vi "ApplyVIPC.vi"(8 "error in (no error)":errorcluster) -> (0 "error out":errorcluster)   [LabVIEW 2020, in "CICD.lvlib"]
doc: "Check currently installed packages and apply specified package if required."
uses:
  CICD.lvlib
  <vilib>/Wiresmith Technology/G CLI/CLI Class/CLI.lvclass
  <vilib>/Wiresmith Technology/G CLI/Argument Parser/Option Set Class/Option Set.lvclass
  <vilib>/Wiresmith Technology/G CLI/Argument Parser/Option Class/Argument Type.ctl
  <vilib>/Wiresmith Technology/G CLI/Argument Parser/Option Class/Option.lvclass
  <vilib>/Wiresmith Technology/G CLI/Argument Parser/Option Class/Option Configuration.ctl
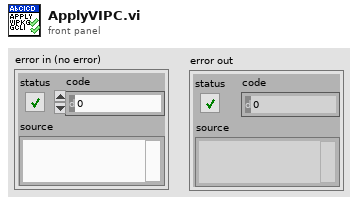
[diagram p1: front panel]
types:
  T1 = typedef "Option Parser.lvlib/Option.lvclass/Option Configuration.ctl" = cluster{"Option Type":T2, "Option Labels":string[], "Key":string, "Description":string, "Required":bool, "Default Value":string}
  T2 = typedef "Option Parser.lvlib/Option.lvclass/Argument Type.ctl" = enum16{"flag", "value"}
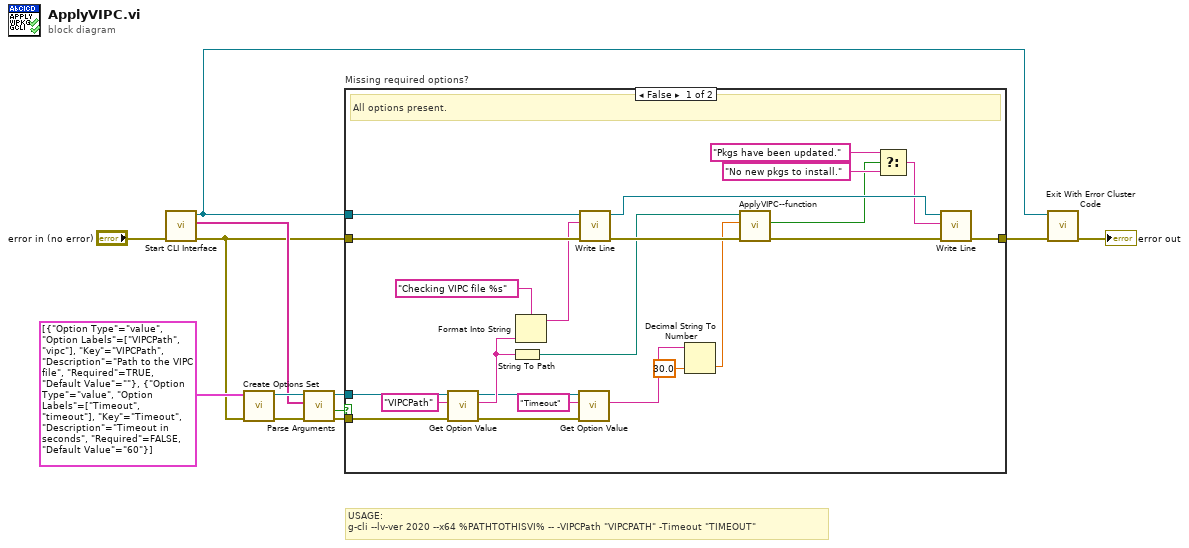
[diagram p0: block diagram]
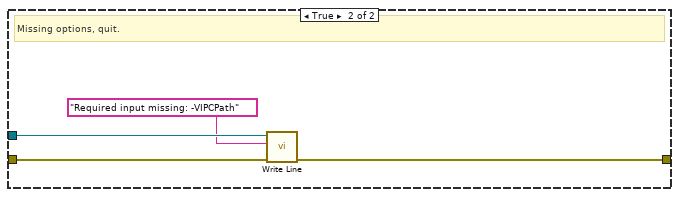
[diagram p2: hidden frame]
diagram:
  # "USAGE:\ng-cli --lv-ver 2020 --x64 %PATHTOTHISVI% -- -VIPCPath \"VIPCPATH\" -Timeout \"TIMEOUT\""
  n1 = call <vilib>:"Start CLI Interface.vi"("error in (no error)"="error in (no error)") -> ("error out"=w4:errorcluster, "Custom Parameters"=w8:string[], "CLI out"=w2:refnum<class "CLI.lvclass">)  [unwired: 7 in, 1 out]
  n2 = call <vilib>:"Create Options Set.vi"("error in (no error)"=w4, "Options"=T1[] [{"Option Type"=enum."value", "Option Labels"=["VIPCPath", "vipc"], "Key"="VIPCPath", "Description"="Path to the VIPC file", "Required"=TRUE, "Default Value"=""}, {"Option Type"=enum."value", "Option Labels"=["Timeout", "timeout"], "Key"="Timeout", "Description"="Timeout in seconds", "Required"=FALSE, "Default Value"="60"}]) -> ("error out"=w10:errorcluster, "Option Set out"=w11:refnum<class "Option Set.lvclass">)  [unwired: 8 in]
  n3 = call <vilib>:"Parse Arguments.vi"("error in (no error)"=w10, "Arguments"=w8, "Option Set in"=w11) -> ("error out"=w6:errorcluster, "Missing Options"=w5:bool, "Option Set out"=w7:refnum<class "Option Set.lvclass">)  [unwired: 5 in, 1 out]
  n4 = case "Missing required options?" shown="False" w5 {
    tunnel: w7 -> [w35 _]
    tunnel: w6 -> [w34 _]
    tunnel: w2 -> [w31 w38]
    tunnel: w4 -> [w32 w39]
    tunnel: [w20 w36] -> w3
    frame False {
      # "All options present."
      n5 = call <vilib>:"Get Option Value.vi"("error in (no error)"=w34, "Option Key"="VIPCPath", "Option Set in"=w35) -> ("error out"=w25:errorcluster, "Value"=w29:string, "Option Set out"=w26:refnum<class "Option Set.lvclass">)  [unwired: 5 in, 1 out]
      n6 = String To Path(string=w29) -> (path=w14:path)
      n7 = Format Into String(format string="Checking VIPC file %s" ("Text to Write"), w29) -> (resulting string=w28:string)  [unwired: 2 in, 1 out]
      n8 = call <vilib>:"Get Option Value.vi"("error in (no error)"=w25, "Option Key"="Timeout", "Option Set in"=w26) -> ("Value"=w22:string)  [unwired: 5 in, 3 out]
      n9 = call <vilib>:"Write Line.vi"("error in (no error)"=w32, "Text to Write"=w28, "CLI in"=w31) -> ("error out"=w27:errorcluster, "CLI out"=w19:refnum<class "CLI.lvclass">)  [unwired: 7 in]
      n10 = Decimal String To Number(string=w22, default (0L)=30.0 ("default (0 I32)")) -> (number=w13:dbl)  [unwired: 1 in, 1 out]
      n11 = call "ApplyVIPC--function.vi"("error in"=w27, "Timeout in seconds"=w13, "VIPC File Path"=w14) -> ("error out"=w21:errorcluster, "Need to Apply?"=w15:bool)  [unwired: 7 in]
      n12 = Select(t="Pkgs have been updated." ("Text to Write"), s=w15, f="No new pkgs to install." ("Text to Write")) -> (s? t:f=w16:string)
      n13 = call <vilib>:"Write Line.vi"("error in (no error)"=w21, "Text to Write"=w16, "CLI in"=w19) -> ("error out"=w20:errorcluster)  [unwired: 7 in, 1 out]
    }
    frame True {
      # "Missing options, quit."
      n14 = call <vilib>:"Write Line.vi"("error in (no error)"=w39, "Text to Write"="Required input missing: -VIPCPath", "CLI in"=w38) -> ("error out"=w36:errorcluster)  [unwired: 7 in, 1 out]
    }
  }
  n15 = call <vilib>:"Exit With Error Cluster Code.vi"("error in (no error)"=w3, "CLI in"=w2) -> ("error out"=→"error out":errorcluster)  [unwired: 9 in]
